vi "SSH_SCP.vi"(6 "Task":enum16{"put", "get", "put folder"}(ring), 7 "scp":cluster{"source":string, "dest":string}, 8 "error in (no error)":errorcluster, 10 "Console In":string, 11 "Python in":cluster{"Python":refnum<k35>, "py file":path}) -> (0 "error out":errorcluster, 2 "Console Out":string, 3 "Python out":cluster{"Python":refnum<k35>, "py file":path})   [LabVIEW 2020]
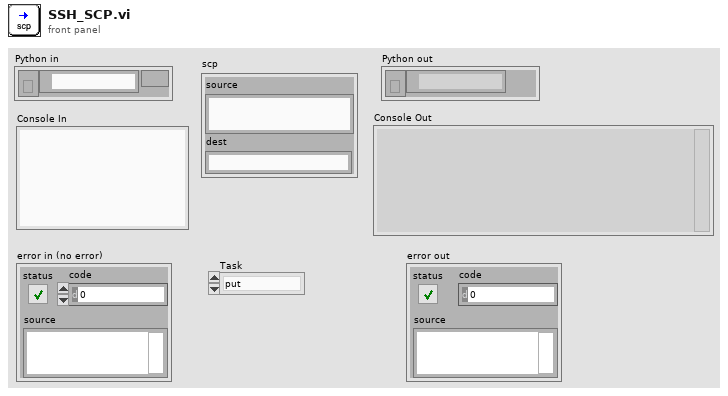
[diagram p1: front panel]
types:
  T1 = cluster{"session out":refnum<k35>, "py file":path}
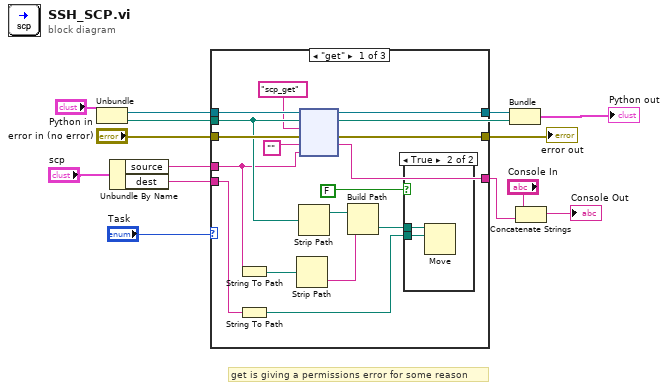
[diagram p0: block diagram]
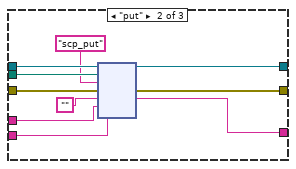
[diagram p3: hidden frame]
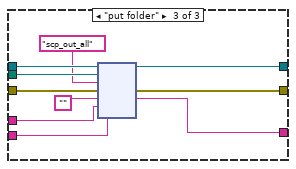
[diagram p4: hidden frame]
diagram:
  # "get is giving a permissions error for some reason"
  n1 = Unbundle("Python in") -> ("Python"=w13:refnum<k35>, "py file"=w7:path)
  n2 = Unbundle By Name("scp") -> ("source"=w6:string, "dest"=w5:string)
  n3 = case shown="\"get\"" "Task" {
    tunnel: [w30 w42 w52] -> w14
    tunnel: w13 -> [w29 w41 w51]
    tunnel: "error in (no error)" -> [w28 w40 w50]
    tunnel: [w27 w39 w49] -> w8
    tunnel: [w17 w33 w43] -> w3
    tunnel: w7 -> [w24 w38 w48]
    tunnel: w6 -> [w23 w37 w47]
    tunnel: w5 -> [w19 w36 w46]
    frame "get" {
      n4 = String To Path(string=w23) -> (path=w22:path)
      n5 = String To Path(string=w19) -> (path=w18:path)
      n6 = Strip Path(path=w22) -> (name=w21:string)  [unwired: 1 out]
      n7 = Strip Path(path=w24) -> (stripped path=w25:path)  [unwired: 1 out]
      n8 = node(w29, w24, "scp_get" ("function name"), w28, "", w23) -> (w30:refnum<k35>, w27:errorcluster, w17:string)  [unwired: 1 in, 2 out]
      n9 = Build Path(base path=w25, name or relative path=w21) -> (appended path=w20:path)
      n10 = case shown="True" FALSE {
        tunnel: w20 -> [_ w32]
        tunnel: w18 -> [_ w31]
        frame False {
        }
        frame True {
          n11 = Move(source path=w32, 10:w31) -> ()  [unwired: 3 in, 3 out]
        }
      }
    }
    frame "put" {
      n12 = node(w41, w38, "scp_put" ("function name"), w40, "", w37, w36) -> (w42:refnum<k35>, w39:errorcluster, w33:string)  [unwired: 2 in, 2 out]
    }
    frame "put folder" {
      n13 = node(w51, w48, "scp_out_all" ("function name"), w50, "", w47, w46) -> (w52:refnum<k35>, w49:errorcluster, w43:string)  [unwired: 2 in, 2 out]
    }
  }
  "error out" <- w8
  n14 = Bundle("session out"=w14, "py file"=w7) -> (→"Python out":T1)  [unwired: 1 in]
  n15 = Concatenate Strings("Console In", w3) -> (→"Console Out":string)
